vi "sadi Write LV.vi"(9 "length":u8, 10 "packet":string, 11 "instance":i32) -> (2 "packet out":string, 3 "function return":u32)   [LabVIEW 2022 SP3, in "SADI_FW3.lvlib"]
doc: "SADI_API_Wrapper unsigned int sadiWrite_LV(int instance,uint8_t *packet, uint8_t length);"
uses:
  SADI_FW3.lvlib
  SADI_FW3.dll
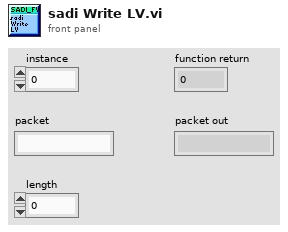
[diagram p1: front panel]
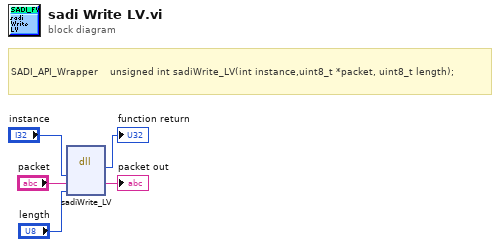
[diagram p0: block diagram]
diagram:
  # "SADI_API_Wrapper    unsigned int sadiWrite_LV(int instance,uint8_t *packet, uint8_t length);"
  n1 = dll-call lib="C:/Users/scer/OneDrive - University of Florida/eml4314c/eml4314Sp24/Resources/release_1_11_24/EML4314c_Sp24_framework_0/LVLib/SADI_FW3.*" fn="sadiWrite_LV"("instance"="instance", "packet"="packet", "length"="length") -> (→"function return":u32, "packet"=→"packet out":string)  [unwired: 5 in, 2 out]
